vi "Get (I16).vi"(8 "error in":errorcluster, 11 "Value in":refnum<class "Value.lvclass">) -> (0 "error out":errorcluster, 1 "Defined?":bool, 2 "Value":i16, 3 "Value out":refnum<class "Value.lvclass">)   [LabVIEW 2019, in "Electronic Datasheet.lvlib" / "Value.lvclass"]
uses:
  Value.lvclass
  Value.lvclass/Value.ctl
  Electronic Datasheet.lvlib
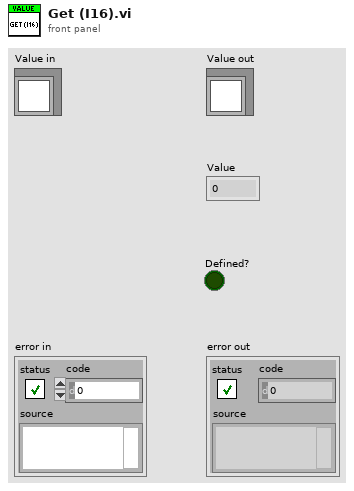
[diagram p1: front panel]
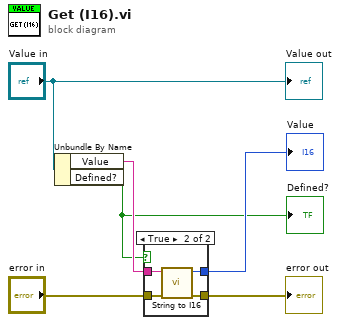
[diagram p0: block diagram]
diagram:
  n1 = Unbundle By Name("Value in") -> ("Value"=w5:string, "Defined?"=w1:bool)
  "Defined?" <- w1
  n2 = case shown="True" w1 {
    tunnel: w5 -> [_ w11]
    tunnel: "error in" -> [w7 w10]
    tunnel: [w7 w9] -> w3
    tunnel: [_ w8] -> w2
    frame False {
    }
    frame True {
      n3 = call "String to I16.vi"("error in"=w10, "Integer String"=w11) -> ("error out"=w9:errorcluster, "I16"=w8:i16)  [unwired: 8 in]
    }
  }
  "error out" <- w3
  "Value" <- w2
  "Value out" <- "Value in"
